vi "Register CycleCompleteEvent.vi"(8 "error in (no error)":errorcluster, 9 "CycleCompleteEvent":refnum<user-event>, 11 "EventManager":refnum<class "EventManager.lvclass">) -> (0 "error out":errorcluster, 1 "EventToken":refnum<class "EventToken.lvclass">, 3 "EventManager out":refnum<class "EventManager.lvclass">)   [LabVIEW 2009]
doc: "Registers an event with the Event Manager. Clients can use the EventHandle to removed events from the Event Manager."
uses:
  EventDataObject/EventData.lvclass
  EventManager.lvclass
  Documents and Settings/Dave/Desktop/Button Latency/trunk/Source/Model/Active Object/EventData Objects/CycleCompleteEventData/CycleCompleteEventData.lvclass
  EventToken/EventToken.lvclass
panel:
  # "See block diagram for more changes."
  # "Do not replace any indicators"
  # "Replace this user event with a user event typed with your event data object.  User events are strictly typed and cannot upcast child objects to parent objects at runtime."
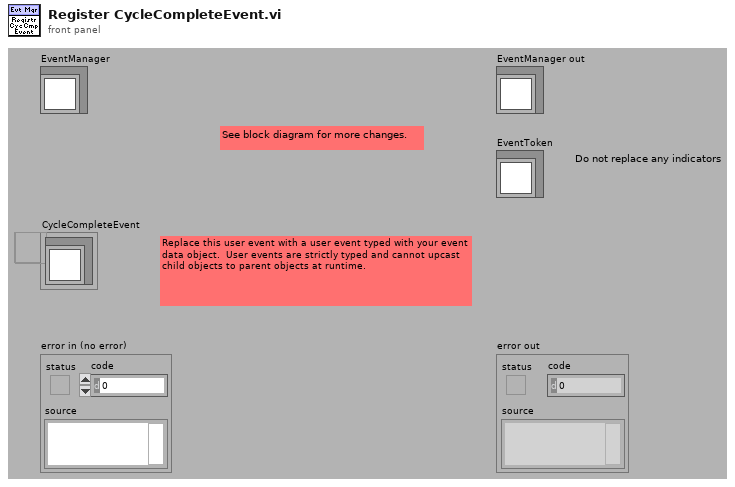
[diagram p1: front panel]
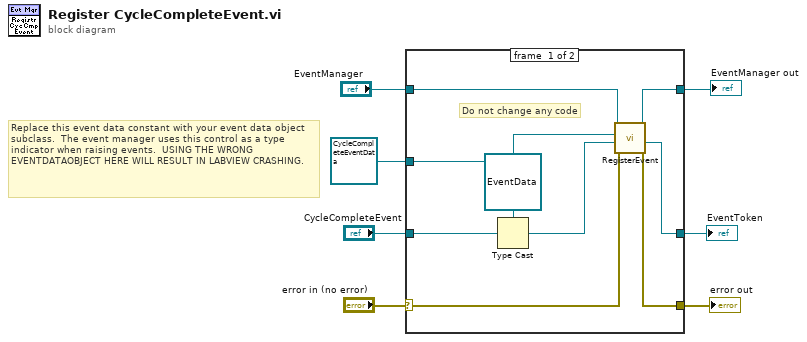
[diagram p0: block diagram]
diagram:
  # "Replace this event data constant with your event data object subclass.  The event manager uses this control as a type indicator when raising events.  USING THE WRONG EVENTDATAOBJECT HERE WILL RESULT IN LABVIEW CRASHING."
  n1 = case shown="No Error" "error in (no error)" {
    selector: "error in (no error)" -> [w10 w18]
    tunnel: [w9 w18] -> w2
    tunnel: "CycleCompleteEvent" -> [w15 _]
    tunnel: refnum<class "CycleCompleteEventData.lvclass"> refnum ("MyEventDataObject") -> [w12 _]
    tunnel: "EventManager" -> [w14 w17]
    tunnel: [w13 w17] -> w6
    tunnel: [w8 _] -> w1
    frame #0 {
      # "Do not change any code"
      n2 = Type Cast(type=refnum<user-event> refnum ("UserEvent"), x=w15) -> (*(type *) &x=w11:refnum<user-event>)
      n3 = call "RegisterEvent.vi"("error in (no error)"=w10, "EventDataUserEvent"=w11, "EventData"=w12, "EventManager in"=w14) -> ("error out"=w9:errorcluster, "EventToken"=w8:refnum<class "EventToken.lvclass">, "EventManager out"=w13:refnum<class "EventManager.lvclass">)  [unwired: 5 out]
    }
    frame #1 {
    }
  }
  "error out" <- w2
  "EventManager out" <- w6
  "EventToken" <- w1
